vi "Init Control.vi"(5 "Group":refnum<class "Group.lvclass">, 6 "Period ms":i64, 7 "VolatusAPI":refnum<class "VolatusAPI.lvclass">, 8 "error in (no error)":errorcluster, 9 "Control MsgQ":refnum<class "MessageQ.lvclass">, 10 "Config Element":refnum<class "Config Element.lvclass">, 11 "Valve in":refnum<class "TimedPWMControl.lvclass">) -> (0 "error out":errorcluster, 3 "Valve out":refnum<class "TimedPWMControl.lvclass">)   [LabVIEW 2020, in "VolatusControl.lvlib" / "TimedPWMControl.lvclass"]
uses:
  TimedPWMControl.lvclass
  lv-cdm/CDM-Config/Config Element/Config Element.lvclass
  Volatus/VolatusAPI/VolatusAPI.lvclass
  Volatus/MessageQ/MessageQ.lvclass
  lv-vecto/Vecto/Group/Group.lvclass
  C:/dev/lv20CE/relink/lv-vecto/Vecto/GroupAbstract/GroupAbstract.lvclass
  lv-control/IG PID/Output Range.ctl
  lv-control/IG PID/Parameters.ctl
  PV Calc.ctl
  TimedPWMControl.lvclass/TimedPWMControl.ctl
  lv-control/IG PID/PID/PID.lvclass
  lv-control/IG PID/IG PID.lvlib
  VolatusControl.lvlib
  lv-vecto/Vecto/GroupAbstract/GroupAbstract.lvclass
  C:/dev/lv20CE/relink/lv-vecto/Vecto/Group/Group.lvclass
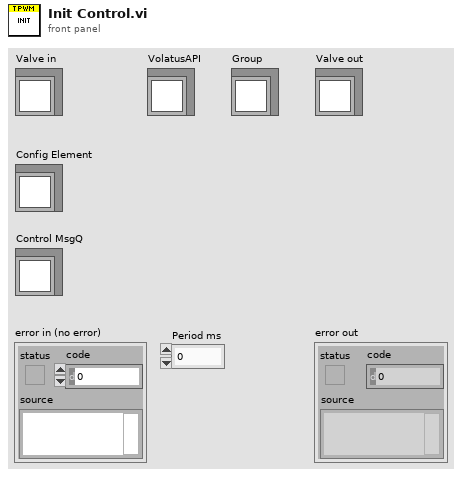
[diagram p1: front panel]
types:
  T1 = typedef "VolatusControl.lvlib/TimedPWMControl.lvclass/PV Calc.ctl" = enum16{"Average", "Median"}
  T2 = typedef "IG PID.lvlib/Parameters.ctl" = cluster{"P Band":dbl, "I Gain":dbl, "D Gain":dbl, "F Gain":dbl}
  T3 = typedef "IG PID.lvlib/Output Range.ctl" = cluster{"Min":dbl, "Max":dbl}
  T4 = typedef "CDM-Config.lvlib/Value Type.ctl" = enum16{"String", "Number", "Bool", "Object", "Array"}
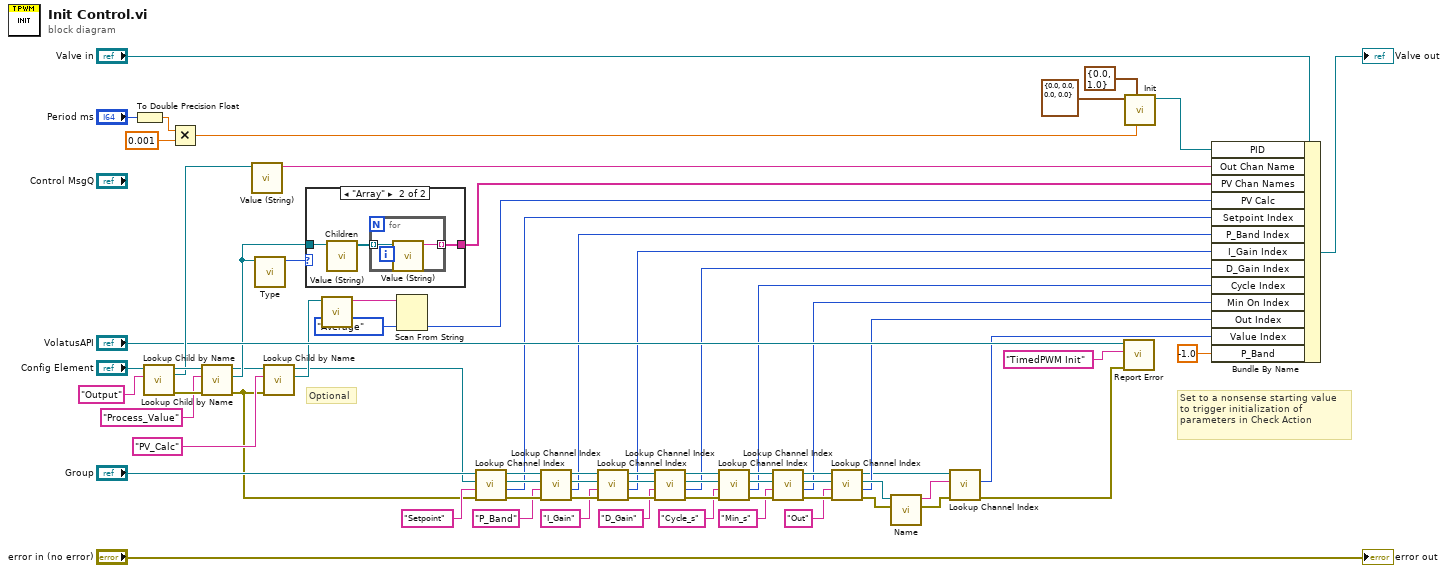
[diagram p0: block diagram]
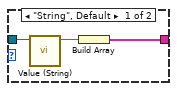
[diagram p2: hidden frame]
diagram:
  # "Optional"
  # "Set to a nonsense starting value to trigger initialization of parameters in Check Action"
  n1 = To Double Precision Float(number="Period ms") -> (double precision float=w3:dbl)
  n2 = call "Lookup Child by Name.vi"("Name"="Output", "Config Element in"="Config Element") -> ("error out"=w71:errorcluster, "Child"=w63:refnum<class "Config Element.lvclass">, "Config Element out"=w65:refnum<class "Config Element.lvclass">)  [unwired: 6 in, 1 out]
  n3 = Multiply(x=w3, y=0.001) -> (x*y=w1:dbl)
  n4 = call "Lookup Child by Name.vi"("error in (no error)"=w71, "Name"="Process_Value", "Config Element in"=w65) -> ("error out"=w9:errorcluster, "Child"=w14:refnum<class "Config Element.lvclass">, "Config Element out"=w12:refnum<class "Config Element.lvclass">)  [unwired: 5 in, 1 out]
  n5 = call "Value (String).vi"("Config Element in"=w63) -> ("String Value"=w58:string)  [unwired: 9 in, 1 out]
  n6 = call "Type.vi"("Config Element in"=w14) -> ("Value Type"=w15:T4)  [unwired: 9 in, 1 out]
  n7 = call "Lookup Child by Name.vi"("error in (no error)"=w9, "Name"="PV_Calc", "Config Element in"=w12) -> ("Child"=w10:refnum<class "Config Element.lvclass">, "Config Element out"=w8:refnum<class "Config Element.lvclass">)  [unwired: 5 in, 2 out]
  n8 = case shown="\"Array\"" w15 {
    tunnel: w14 -> [w74 w77]
    tunnel: [w72 w75] -> w13
    frame "String", Default {
      n9 = call "Value (String).vi"("Config Element in"=w74) -> ("String Value"=w73:string)  [unwired: 9 in, 1 out]
      n10 = Build Array(w73) -> (w72:string[])
    }
    frame "Array" {
      n11 = call "Children.vi"("Config Element in"=w77) -> ("Elements"=w76:refnum<class "Config Element.lvclass">[])  [unwired: 9 in, 1 out]
      n12 = for {
        tunnel: w76 -> [w79] mode=indexing
        tunnel: [w78] -> w75 mode=indexing
        n13 = call "Value (String).vi"("Config Element in"=w79) -> ("String Value"=w78:string)  [unwired: 9 in, 1 out]
      }
    }
  }
  n14 = call "Value (String).vi"("Config Element in"=w10) -> ("String Value"=w7:string)  [unwired: 9 in, 1 out]
  n15 = Scan From String(input string=w7, default 1=PV_Calc."Average" ("PV Calc")) -> (output 1=w5:T1)  [unwired: 3 in, 3 out]
  n16 = call "Lookup Channel Index.vi"("error in (no error)"=w9, "Meta Value"="Setpoint" ("Name"), "Config Element in"=w8, "Group in"="Group") -> ("error out"=w53:errorcluster, "Index"=w23:i32, "Config Element"=w54:refnum<class "Config Element.lvclass">, "Group"=w55:refnum<class "Group.lvclass">)  [unwired: 4 in]
  n17 = call "Lookup Channel Index.vi"("error in (no error)"=w53, "Meta Value"="P_Band" ("Name"), "Config Element in"=w54, "Group in"=w55) -> ("error out"=w51:errorcluster, "Index"=w24:i32, "Config Element"=w50:refnum<class "Config Element.lvclass">, "Group"=w49:refnum<class "Group.lvclass">)  [unwired: 4 in]
  n18 = call "Lookup Channel Index.vi"("error in (no error)"=w51, "Meta Value"="I_Gain" ("Name"), "Config Element in"=w50, "Group in"=w49) -> ("error out"=w45:errorcluster, "Index"=w25:i32, "Config Element"=w46:refnum<class "Config Element.lvclass">, "Group"=w47:refnum<class "Group.lvclass">)  [unwired: 4 in]
  n19 = call "Lookup Channel Index.vi"("error in (no error)"=w45, "Meta Value"="D_Gain" ("Name"), "Config Element in"=w46, "Group in"=w47) -> ("error out"=w43:errorcluster, "Index"=w26:i32, "Config Element"=w42:refnum<class "Config Element.lvclass">, "Group"=w41:refnum<class "Group.lvclass">)  [unwired: 4 in]
  n20 = call "Lookup Channel Index.vi"("error in (no error)"=w43, "Meta Value"="Cycle_s" ("Name"), "Config Element in"=w42, "Group in"=w41) -> ("error out"=w37:errorcluster, "Index"=w27:i32, "Config Element"=w38:refnum<class "Config Element.lvclass">, "Group"=w39:refnum<class "Group.lvclass">)  [unwired: 4 in]
  n21 = call "Lookup Channel Index.vi"("error in (no error)"=w37, "Meta Value"="Min_s" ("Name"), "Config Element in"=w38, "Group in"=w39) -> ("error out"=w33:errorcluster, "Index"=w28:i32, "Config Element"=w34:refnum<class "Config Element.lvclass">, "Group"=w35:refnum<class "Group.lvclass">)  [unwired: 4 in]
  n22 = call "Lookup Channel Index.vi"("error in (no error)"=w33, "Meta Value"="Out" ("Name"), "Config Element in"=w34, "Group in"=w35) -> ("error out"=w31:errorcluster, "Index"=w29:i32, "Config Element"=w30:refnum<class "Config Element.lvclass">, "Group"=w21:refnum<class "Group.lvclass">)  [unwired: 4 in]
  n23 = call "Name.vi"("error in (no error)"=w31, "Config Element in"=w30) -> ("error out"=w19:errorcluster, "Name"=w20:string)  [unwired: 8 in]
  n24 = call "Lookup Channel Index.vi"("error in (no error)"=w19, "Channel Name"=w20, "GroupAbstract in"=w21) -> ("error out"=w17:errorcluster, "Index"=w18:i32)  [unwired: 6 in, 1 out]
  n25 = call "Report Error.vi"("error in (no error)"=w17, "Context"="TimedPWM Init", "VolatusAPI in"="VolatusAPI") -> ()  [unwired: 7 in, 2 out]
  n26 = call "Init.vi"("dT (Auto)"=w1, "Output Range"=T3 {"Min"=0.0, "Max"=1.0}, "Parameters"=T2 {"P Band"=0.0, "I Gain"=0.0, "D Gain"=0.0, "F Gain"=0.0}) -> ("PID out"=w62:refnum<class "PID.lvclass">)  [unwired: 7 in, 1 out]
  n27 = Bundle By Name(cluster="Valve in", "PID"=w62, "Out Chan Name"=w58, "PV Chan Names"=w13, "PV Calc"=w5, "Setpoint Index"=w23, "P_Band Index"=w24, "I_Gain Index"=w25, "D_Gain Index"=w26, "Cycle Index"=w27, "Min On Index"=w28, "Out Index"=w29, "Value Index"=w18, "P_Band"=-1.0) -> (→"Valve out":refnum<class "TimedPWMControl.lvclass">)
  "error out" <- "error in (no error)"
